vi "Select Target Circle Colors.vi"(1 "USB cameras":i32, 2 "Image client connect errors":errorcluster[](array[cluster])) -> (0 "Array":u32[](array[numeric]))   [LabVIEW 2013]
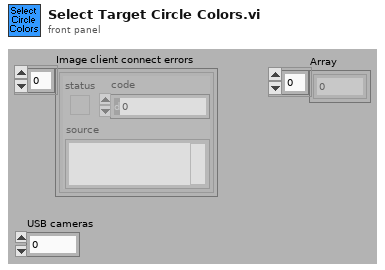
[diagram p1: front panel]
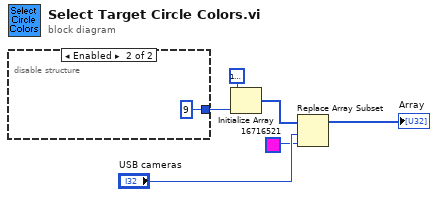
[diagram p0: block diagram]
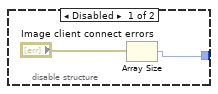
[diagram p2: hidden frame]
diagram:
  n1 = disable-structure shown="Enabled" {
    disable-tunnel: [w8 9] -> w2
    frame Disabled {
      n2 = Array Size(array="Image client connect errors") -> (size(s)=w8:i32)
    }
    frame Enabled {
    }
  }
  n3 = Initialize Array(u32 16777222 ("Color"), w2) -> (w3:u32[])
  n4 = Replace Array Subset(array=w3, new element=u32 16716521 ("Color"), index="USB cameras") -> (→"Array":u32[])
